vi "KML-dataParse.vi"(0 "data in":string) -> (1 "ALT":string, 3 "Cur loc (out)":string)   [LabVIEW 8.6]
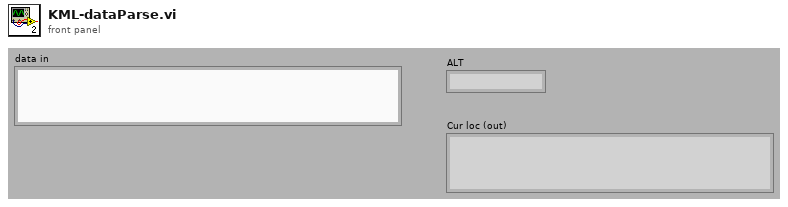
[diagram p1: front panel]
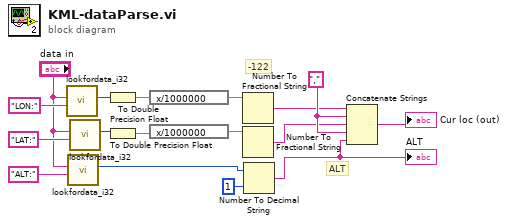
[diagram p0: block diagram]
diagram:
  w17 = ","
  # "-122"
  # "ALT"
  n1 = call "lookfordata_i32.vi"("string (in)"="data in", "Header"="LON:") -> ("output number"=w11:i32)  [unwired: 4 in, 2 out]
  n2 = call "lookfordata_i32.vi"("string (in)"="data in", "Header"="ALT:" ("regular expression")) -> ("output number"=w3:i32)  [unwired: 4 in, 2 out]
  n3 = call "lookfordata_i32.vi"("string (in)"="data in", "Header"="LAT:") -> ("output number"=w10:i32)  [unwired: 4 in, 2 out]
  n4 = To Double Precision Float(number=w11) -> (double precision float=w12:dbl)
  n5 = To Double Precision Float(number=w10) -> (double precision float=w9:dbl)
  n6 = expression code="x/1000000"(w12) -> (w8:dbl)
  n7 = expression code="x/1000000"(w9) -> (w7:dbl)
  n8 = Number To Fractional String(number=w8) -> (F-format string=w5:string)  [unwired: 3 out]
  n9 = Number To Fractional String(number=w7) -> (F-format string=w4:string)  [unwired: 3 out]
  n10 = Number To Decimal String(number=w3, width (-)=i16 1) -> (decimal integer string=w2:string)
  "ALT" <- w2
  n11 = Concatenate Strings(w5, w17, w4, w17, w2) -> (→"Cur loc (out)":string)
